vi "I-SRC Shutdown (Poly).vi"   [LabVIEW 2016, in "Hall Effect Library.lvlib"]
uses:
  Hall Effect Library.lvlib
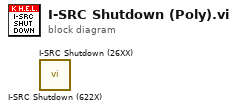
[diagram p0: block diagram]
diagram:
  n1 = call "I-SRC Shutdown (622X).vi"() -> ()  [unwired: 10 in, 2 out]
  n2 = call "I-SRC Shutdown (26XX).vi"() -> ()  [unwired: 10 in, 2 out]
